vi "Configure Multi Eval Meas Power Vs Time Limit.vi"(7 "Power Limits (On)":bool=TRUE, 8 "error in (no error)":errorcluster, 9 "Average Power (0)":dbl format="%^.3e", 10 "Instance (1)":i32=1, 11 "VISA resource name":refnum<visa-resource-name>) -> (0 "error out":errorcluster, 3 "VISA resource name out":refnum<visa-resource-name>)   [LabVIEW 2015, in "Rohde&Schwarz CMP LR WPAN Measurement.lvlib"]
doc: "Sets and enables or disables a lower limit for PVT measurements.\n\nOrder of parameters:\n<AveragePower>\n<AvgPowEnabled>\n\nAttribute:\n-\n\nRemote-control command:\nCONFigure:WPAN:MEAS<i>:MEValuation:LIMit:PVTime"
uses:
  <instrlib>/Rohde&Schwarz CMP LR WPAN Measurement/Rohde&Schwarz CMP LR WPAN Measurement.lvlib
  <instrlib>/Rohde&Schwarz CMP LR WPAN Measurement/Private/rsidr_core.llb/rsidr_core.lvlib
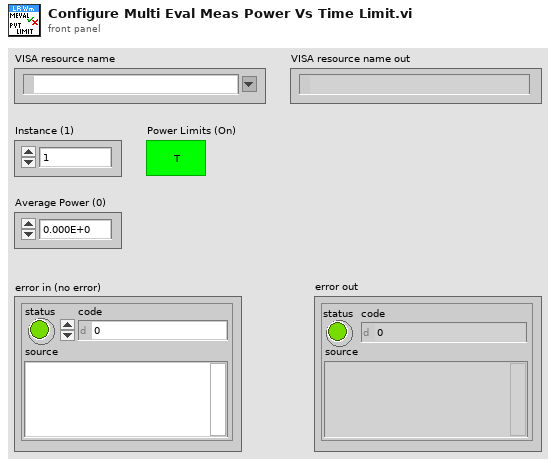
[diagram p1: front panel]
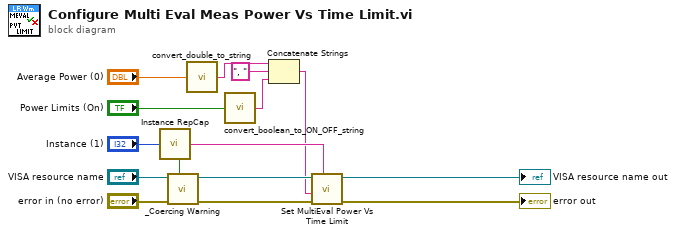
[diagram p0: block diagram]
diagram:
  n1 = call <instrlib>:"Instance RepCap.vi"("Instance In"="Instance (1)") -> ("In Range?"=w15:bool, "RepCap Identifier Out"=w9:string)  [unwired: 1 in]
  n2 = call <instrlib>:"_Coercing Warning.vi"("In Range?"=w15, "error in (no error)"="error in (no error)", "VISA resource name"="VISA resource name") -> ("error out"=w6:errorcluster, "VISA resource name out"=w5:refnum<visa-resource-name>)  [unwired: 7 in]
  n3 = call <instrlib>:"convert_double_to_string.vi"("double in"="Average Power (0)") -> ("string out"=w12:string)  [unwired: 4 in]
  n4 = call <instrlib>:"convert_boolean_to_ON_OFF_string.vi"("boolean value in"="Power Limits (On)") -> ("string value out"=w10:string)  [unwired: 4 in]
  n5 = Concatenate Strings(w12, ", " ("string"), w10) -> (w2:string)
  n6 = call "Set MultiEval Power Vs Time Limit"("Repeated Capabilities"=w9, "error in (no error)"=w6, "MultiEval Power Vs Time Limit ()"=w2, "instrument handle"=w5) -> ("error out"=→"error out":errorcluster, "instrument handle out"=→"VISA resource name out":refnum<visa-resource-name>)  [unwired: 6 in]
